vi "Step Update All.vi"(8 "error in (no error)":errorcluster, 10 "Steps":T2[](array[typedef]), 11 "Connection Refnum":T1) -> (0 "error out":errorcluster, 3 "Connection Refnum":T1)   [LabVIEW 2011]
uses:
  Step Record.ctl
  SI.LIB/ODBC/SQL Controls/Connection Refnum.ctl
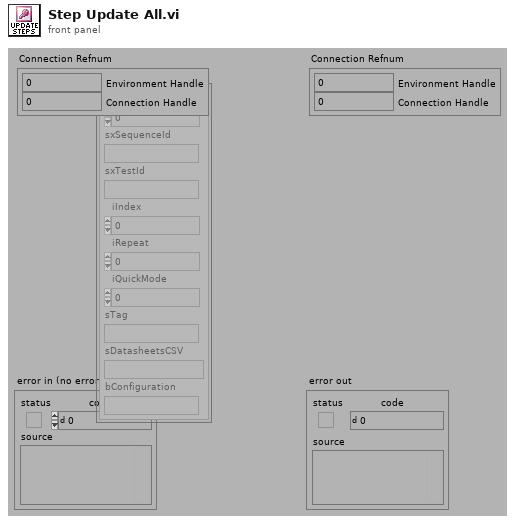
[diagram p1: front panel]
types:
  T1 = typedef "Connection Refnum.ctl" = cluster{"Environment Handle":i32, "Connection Handle":i32}
  T2 = typedef "Step Record.ctl" = cluster{"ixStep":i32, "sxSequenceId":string, "sxTestId":string, "iIndex":i32, "iRepeat":i32, "iQuickMode":i32, "sTag":string, "sDatasheetsCSV":string, "bConfiguration":string}
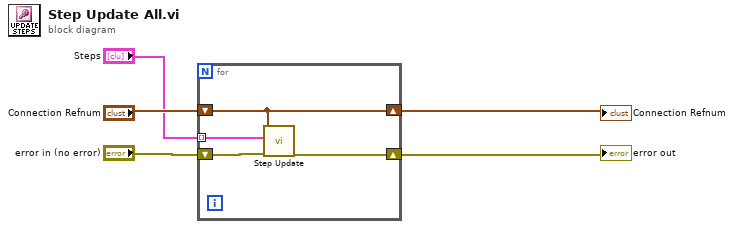
[diagram p0: block diagram]
diagram:
  n1 = for {
    shift-right: [w8] -> w3
    shift-left: "Connection Refnum" -> [w8]
    tunnel: "Steps" -> [w9] mode=indexing
    shift-right: [w6] -> w1
    shift-left: "error in (no error)" -> [w7]
    n2 = call "Step Update.vi"("error in (no error)"=w7, "Step Record (empty)"=w9, "Connection Refnum"=w8) -> ("error out"=w6:errorcluster)  [unwired: 8 out]
  }
  "error out" <- w1
  "Connection Refnum" <- w3
